vi "GetFrontPanel.vi"(8 "Error In":errorcluster, 11 "object in":refnum<class "HeaderTriekselSoft.lvclass">) -> (0 "Error Out":errorcluster, 2 "FrontPanel":refnum<class "FrontPanelControl.lvclass">, 3 "object out":refnum<class "HeaderTriekselSoft.lvclass">)   [LabVIEW 2021, in "HeaderTriekselSoft.lvclass"]
doc: "Retrieve the FrontPanelControl for controlling the state of the user interface front panel"
uses:
  HeaderTriekselSoft.lvclass
  .Externals/Library_UserInterface_FrontPanelControl/FrontPanelControl/FrontPanelControl.lvclass
  HeaderTriekselSoft.lvclass/HeaderTriekselSoft.ctl
panel:
  # "TriekselSoft"
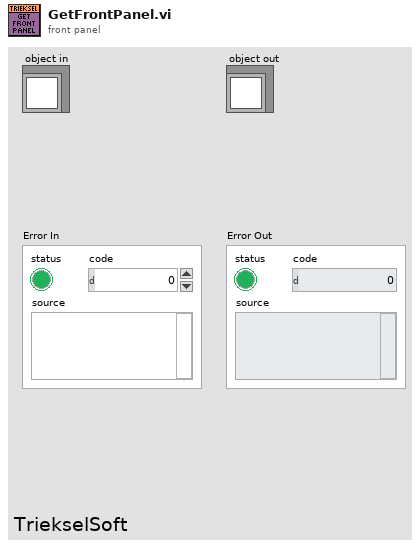
[diagram p1: front panel]
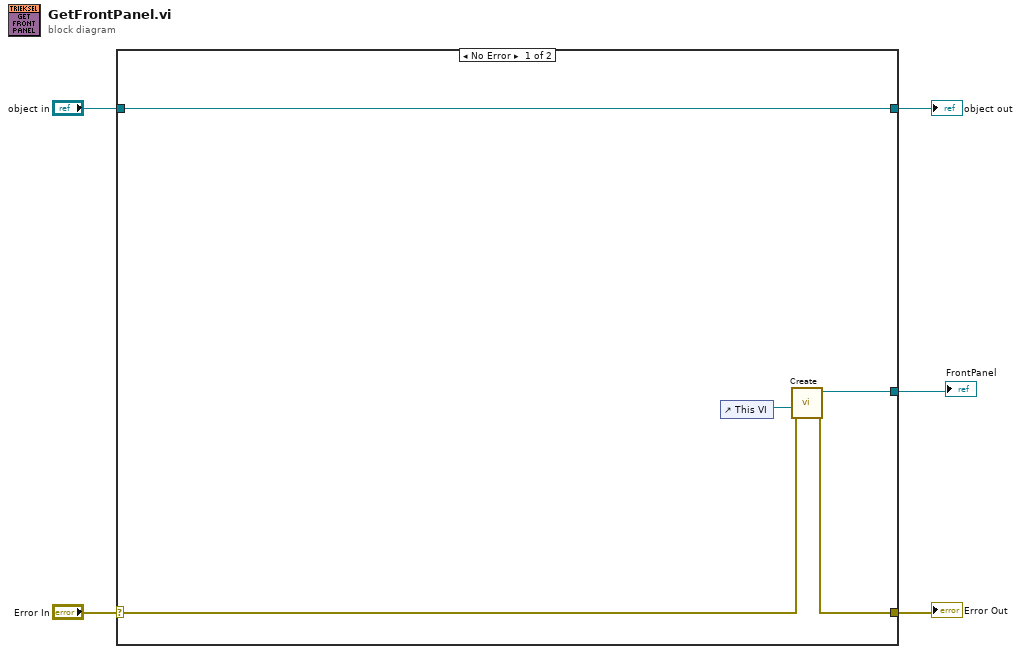
[diagram p0: block diagram]
diagram:
  n1 = case shown="No Error" "Error In" {
    selector: "Error In" -> [w8 w12]
    tunnel: [w7 w12] -> w4
    tunnel: [w10 w11] -> w2
    tunnel: "object in" -> [w10 w11]
    tunnel: [w6 _] -> w1
    frame No Error {
      n2 = control-ref of="This VI"() -> (w9:refnum<vi>)
      n3 = call "Create.vi"("ErrorIn"=w8, "VIRef"=w9) -> ("ErrorOut"=w7:errorcluster, "ObjectOut"=w6:refnum<class "FrontPanelControl.lvclass">)  [unwired: 8 in]
    }
    frame Error {
    }
  }
  "Error Out" <- w4
  "object out" <- w2
  "FrontPanel" <- w1
